vi "Flang Teleop.vi"(9 "Driver Buttons":bool[](array[boolean]), 11 "Driver Axes":dbl[](array[numeric])) -> ()   [LabVIEW 2019]
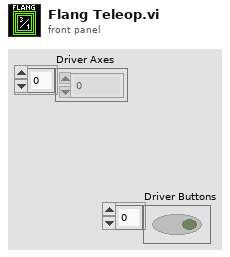
[diagram p1: front panel]
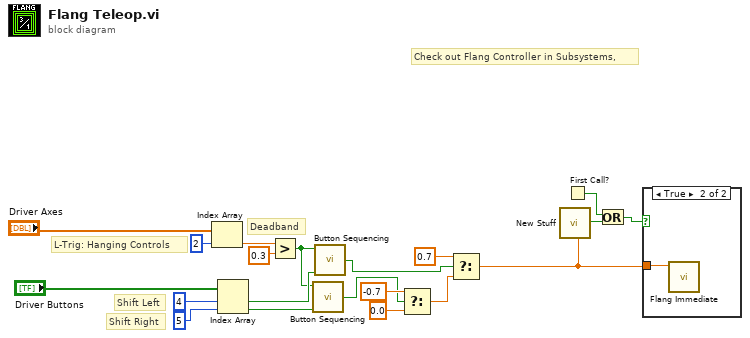
[diagram p0: block diagram]
diagram:
  # "Deadband"
  # "L-Trig: Hanging Controls"
  # "Shift Right"
  # "Shift Left"
  # "Check out Flang Controller in Subsystems,"
  n1 = Index Array(array="Driver Axes", index=2) -> (element=w10:dbl)
  n2 = Index Array(array="Driver Buttons", index #1=4 ("index"), index #2=5 ("index")) -> (element #1=w8:bool, element #2=w6:bool)
  n3 = Greater?(x=w10, y=0.3) -> (0:w7:bool)
  n4 = call "Button Sequencing.vi"("2"=w6, "1"=w7) -> ("Boolean"=w4:bool)  [unwired: 4 in]
  n5 = call "Button Sequencing.vi"("2"=w8, "1"=w7) -> ("Boolean"=w5:bool)  [unwired: 4 in]
  n6 = Select(t=-0.7, s=w4, f=0.0) -> (s? t:f=w17:dbl)
  n7 = Select(t=0.7, s=w5, f=w17) -> (s? t:f=w20:dbl)
  n8 = call "New Stuff.vi"("Variant 9"=w20) -> ("x != y?"=w3:bool)  [unwired: 26 in]
  n9 = First Call?() -> (First Call?: T/F=w1:bool)
  n10 = Or(x=w1, y=w3) -> (x .or. y?=w2:bool)
  n11 = case shown="True" w2 {
    tunnel: w20 -> [_ w21]
    frame False {
    }
    frame True {
      n12 = call "Flang Immediate.vi"("Pole Runner"=w21) -> ()  [unwired: 10 in, 1 out]
    }
  }
